vi "DSF.Memory.Pointer.U16.New.vi"(8 "error in (no error)":errorcluster, 11 "count (1)":u64 format="%d elements") -> (0 "error out":errorcluster, 3 "pointer":refnum<class "DSF.Memory.Pointer.U16.lvclass">)   [LabVIEW 2016, in "DSF.Memory.lvlib" / "DSF.Memory.Pointer.U16.lvclass"]
uses:
  DSF.Memory.Pointer.U16.lvclass
  C:/Git/SourceTree/data-sharing-framework/Source/Submodules/Memory Manager/Source/Classes/Pointer.Internal/Memory.Pointer.Internal.lvclass
  Submodules/Memory Manager/Source/Classes/Pointer.Internal/Memory.Pointer.Internal.lvclass
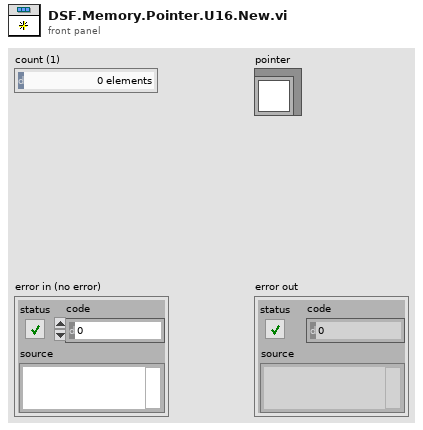
[diagram p1: front panel]
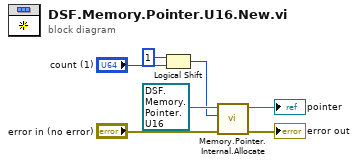
[diagram p0: block diagram]
diagram:
  n1 = Logical Shift(y=i16 1 ("power of 2"), x="count (1)") -> (x << y=w1:u64)
  n2 = call "Memory.Pointer.Internal.Allocate.vi"("error in (no error)"="error in (no error)", "size"=w1, "pointer in"=refnum<class "DSF.Memory.Pointer.U16.lvclass"> refnum ("DBL Pointer")) -> ("error out"=→"error out":errorcluster, "pointer out"=→"pointer":refnum<class "DSF.Memory.Pointer.U16.lvclass">)  [unwired: 7 in]
